vi "set tuner if gain.vi"(8 "error in (no error)":errorcluster, 9 "Gain (dB)":dbl, 10 "Stage":i32, 11 "DeviceRefnum":u64) -> (0 "error out":errorcluster, 2 "function return":i32, 3 "DeviceRefnum Out":u64)   [LabVIEW 2015, in "rtlsdr.lvlib"]
doc: "Set the intermediate frequency gain for the device."
uses:
  rtlsdr.lvlib
  rtlsdr/rtlsdr.dll
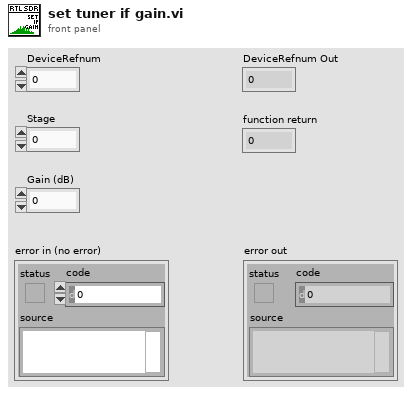
[diagram p1: front panel]
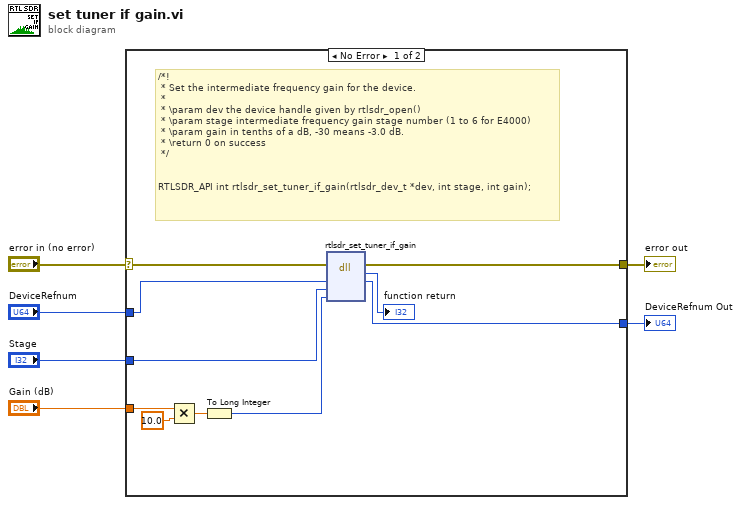
[diagram p0: block diagram]
diagram:
  n1 = case shown="No Error" "error in (no error)" {
    selector: "error in (no error)" -> [w8 w18]
    tunnel: "Stage" -> [w15 _]
    tunnel: "DeviceRefnum" -> [w14 w17]
    tunnel: [w13 w17] -> w4
    tunnel: "Gain (dB)" -> [w12 _]
    tunnel: [w7 w18] -> w1
    frame No Error {
      # "/*!\n * Set the intermediate frequency gain for the device.\n *\n * \\param dev the device handle given by rtlsdr_open()\n * \\param stage intermediate frequency gain stage number (1 to 6 for E4000)\n * \\param gain in tenths of a dB, -30 means -3.0 dB.\n * \\return 0 on success\n */\n\n\nRTLSDR_API int rtlsdr_set_tuner_if_gain(rtlsdr_dev_t *dev, int stage, int gain);"
      n2 = Multiply(x=w12, y=10.0) -> (x*y=w10:dbl)
      n3 = To Long Integer(number=w10) -> (32bit integer=w9:i32)
      n4 = dll-call lib="C:/Users/TheDoctor/Documents/Projects/Labview Libraries/rtlsdr/rtlsdr.*" fn="rtlsdr_set_tuner_if_gain"(error in=w8, "DeviceRefnum"=w14, "Stage"=w15, "Gain"=w9) -> (error out=w7:errorcluster, "return type"=→"function return":i32, "DeviceRefnum"=w13:u64)  [unwired: 4 in, 1 out]
    }
    frame Error {
    }
  }
  "DeviceRefnum Out" <- w4
  "error out" <- w1
